vi "CreatMessageSection.vi"(0 "Port_No.":refnum<k21>, 2 "MessageFrame":refnum<k21>, 5 "错误输入（无错误）":errorcluster) -> (14 "session out":refnum<k21>, 15 "Sigs":refnum<k21>[](array[refnum]), 19 "error out":errorcluster)   [LabVIEW 2020]
uses:
  <vilib>/xnet/xnet.llb/XNET Create Session (Signal Output Single-point).vi
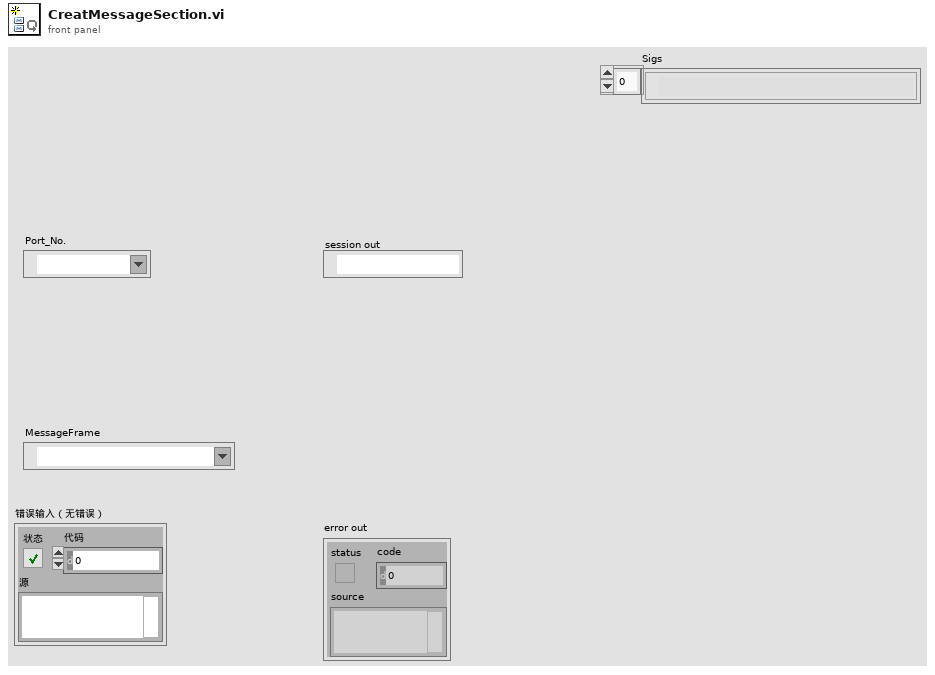
[diagram p1: front panel]
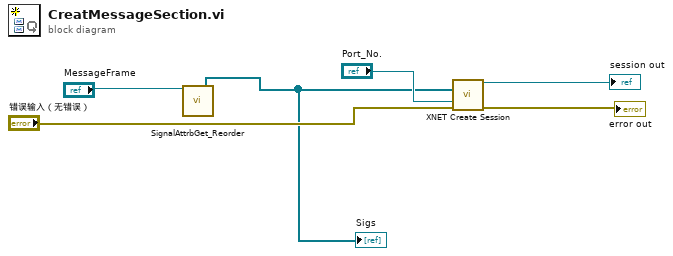
[diagram p0: block diagram]
diagram:
  n1 = call "SignalAttrbGet_Reorder.vi"("MessageFrame"="MessageFrame") -> ("SignalArryOderByStartBit"=w2:refnum<k21>[])  [unwired: 12 in, 6 out]
  "Sigs" <- w2
  n2 = call-poly <vilib>:"XNET Create Session.vi"("signal list"=w2, "interface"="Port_No.", "error in (no error)"="错误输入（无错误）") -> ("session out"=→"session out":refnum<k21>, "error out"=→"error out":errorcluster)  [unwired: 11 out]
